vi "Find Millennia V.vi"(8 "error in (no error)":errorcluster, 11 "VISA resource name":refnum<visa-resource-name>="COM1") -> (0 "error out":errorcluster, 2 "Millennia V found":bool, 3 "VISA resource name out":refnum<visa-resource-name>="COM1")   [LabVIEW 2017, in "Millennia V.lvclass"]
doc: "Checks the given port for the Millennia V laser."
uses:
  Millennia V.lvclass
  <vilib>/Instr/_visa.llb/VISA Configure Serial Port (Instr).vi
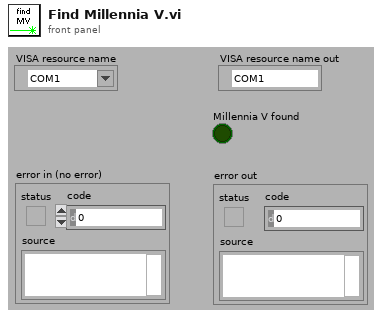
[diagram p1: front panel]
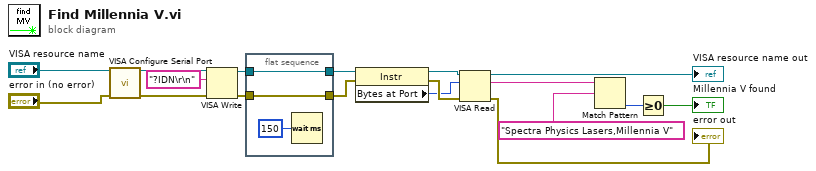
[diagram p0: block diagram]
diagram:
  n1 = call-poly "VISA Configure Serial Port"("VISA resource name"="VISA resource name", "error in (no error)"="error in (no error)") -> ("VISA resource name out"=w13:refnum<visa-resource-name>, "error out"=w12:errorcluster)  [unwired: 12 in]
  n2 = VISA Write(VISA resource name=w13, write buffer="?IDN\r\n", error in (no error)=w12) -> (VISA resource name out=w16:refnum<visa-resource-name>, error out=w15:errorcluster)  [unwired: 1 out]
  n3 = flat-sequence {
    tunnel: w15 -> [w19]
    tunnel: w16 -> [w20]
    tunnel: [w20] -> w9
    tunnel: [w19] -> w8
    frame #0 {
      n4 = Wait (ms)(milliseconds to wait=u32 150) -> ()  [unwired: 1 out]
    }
  }
  n5 = property class="Instr"(reference=w9, error in=w8) -> (error out=w11:errorcluster, "Bytes at Port"=w10:u32)  [unwired: 1 out]
  n6 = VISA Read(VISA resource name=w9, byte count=w10, error in (no error)=w11) -> (VISA resource name out=→"VISA resource name out":refnum<visa-resource-name>, read buffer=w7:string, error out=→"error out":errorcluster)  [unwired: 1 out]
  n7 = Match Pattern(string=w7, regular expression="Spectra Physics Lasers,Millennia V") -> (offset past match=w5:i32)  [unwired: 1 in, 3 out]
  n8 = Greater Or Equal To 0?(x=w5) -> (x >= 0?=→"Millennia V found":bool)
